vi "DAQ.vi"(8 "error in":errorcluster, 11 "Baseline Mocon \npiD-Tech plus in":refnum<class "Baseline Mocon piD-Tech plus.lvclass">) -> (0 "error out":errorcluster, 2 "Data":dbl[](array[numeric]), 3 "Baseline Mocon \npiD-Tech plus out":refnum<class "Baseline Mocon piD-Tech plus.lvclass">)   [LabVIEW 2011, in "Baseline Mocon piD-Tech plus.lvclass"]
uses:
  Baseline Mocon piD-Tech plus.lvclass
  Baseline Mocon piD-Tech plus.lvclass/Baseline Mocon piD-Tech plus.ctl
  <vilib>/DAQmx/read.llb/DAQmx Read (Analog DBL 1Chan 1Samp).vi
  <vilib>/DAQmx/miscellaneous.llb/DAQmx Fill In Error Info.vi
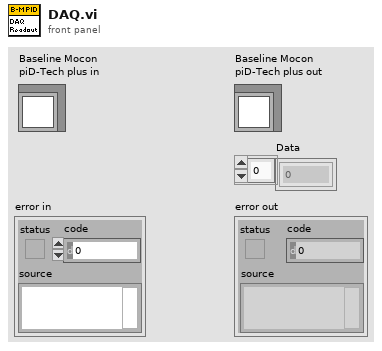
[diagram p1: front panel]
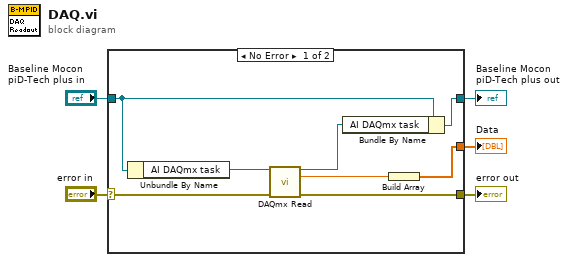
[diagram p0: block diagram]
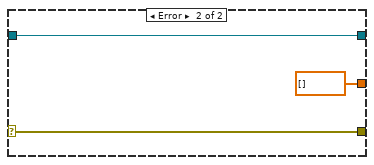
[diagram p2: hidden frame]
diagram:
  n1 = case shown="No Error" "error in" {
    selector: "error in" -> [w12 w16]
    tunnel: [w8 w16] -> w4
    tunnel: [w7 w15] -> w2
    tunnel: "Baseline Mocon \npiD-Tech plus in" -> [w11 w15]
    tunnel: [w6 dbl[] []] -> w1
    frame No Error {
      n2 = Unbundle By Name(w11) -> ("AI DAQmx task"=w13:refnum<k21>)
      n3 = call-poly <vilib>:"DAQmx Read.vi"("task/channels in"=w13, "error in"=w12) -> ("task out"=w10:refnum<k21>, "data"=w9:dbl, "error out"=w8:errorcluster)  [unwired: 11 in]
      n4 = Bundle By Name(cluster=w11, "AI DAQmx task"=w10) -> (w7:refnum<class "Baseline Mocon piD-Tech plus.lvclass">)
      n5 = Build Array(w9) -> (w6:dbl[])
    }
    frame Error {
    }
  }
  "error out" <- w4
  "Baseline Mocon \npiD-Tech plus out" <- w2
  "Data" <- w1
